vi "FILTR1.vi"() -> ()   [LabVIEW 2018]
panel:
  out "read buffer 2":string
  out "read buffer":string
  out "Postep %":dbl format="%#_2g"
  in  "START":i32=100
  in  "STOP":i32=1000
  out "XY Graph":cluster{"X":dbl[], "Y":dbl[]}[](graph)
  out "CHAN2VRMS":string
  out "CHAN1 VRMS":string
  in  "Step":i32=100
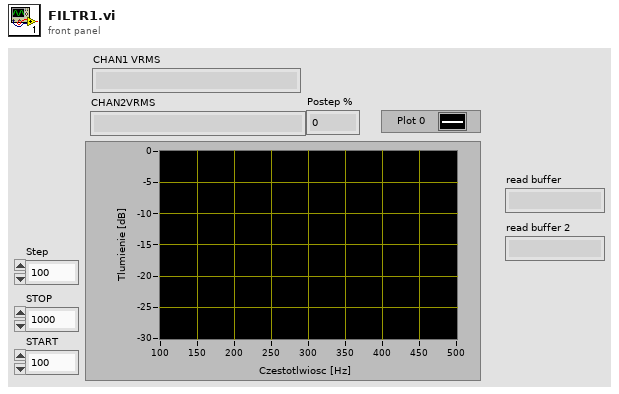
[diagram p1: front panel]
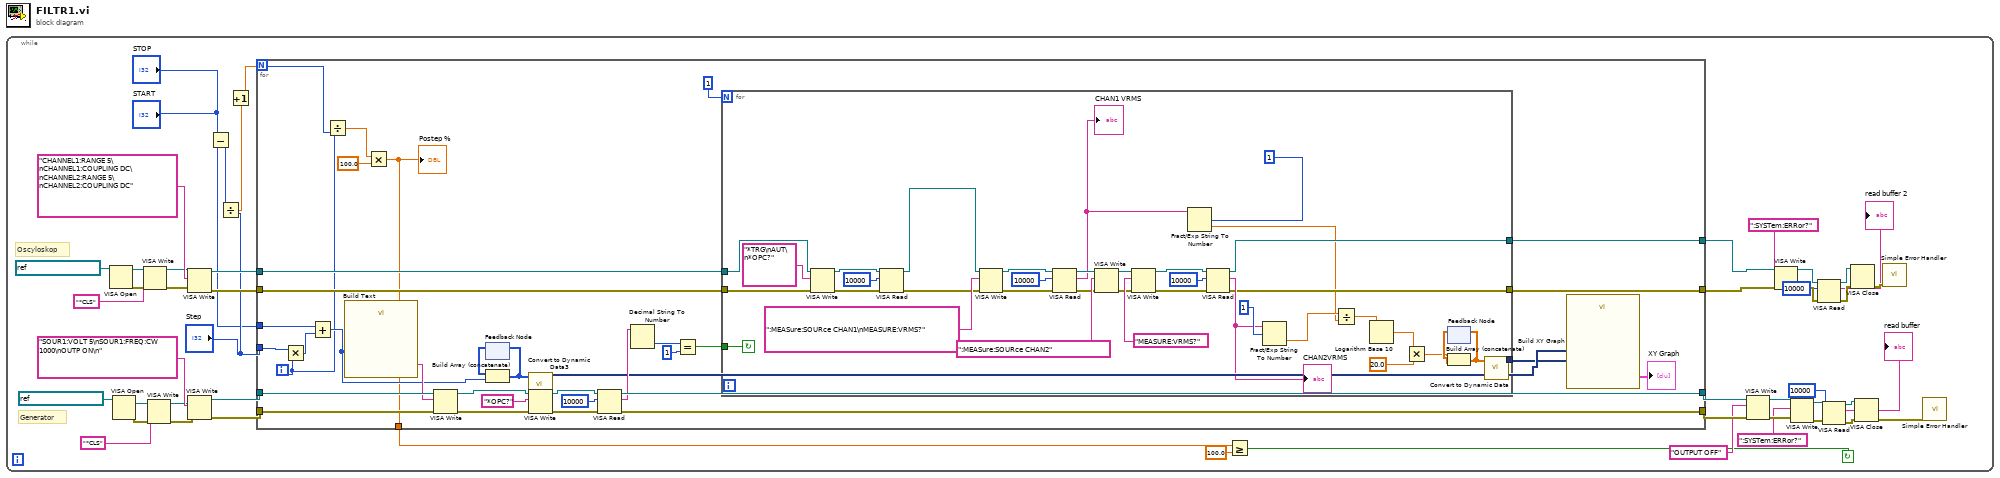
[diagram p0: block diagram]
diagram:
  n1 = while {
    stop <- w29 continue-if-true
    # "Generator"
    # "Oscyloskop"
    n2 = VISA Open(VISA resource name=refnum<visa-resource-name> "GPIB0::1::INSTR") -> (VISA resource name=w25:refnum<visa-resource-name>, error out=w28:errorcluster)  [unwired: 4 in]
    n3 = VISA Open(VISA resource name=refnum<visa-resource-name> "GPIB0::2::INSTR") -> (VISA resource name=w21:refnum<visa-resource-name>, error out=w20:errorcluster)  [unwired: 4 in]
    n4 = VISA Write(VISA resource name=w25, write buffer="*CLS", error in (no error)=w28) -> (VISA resource name out=w26:refnum<visa-resource-name>, error out=w27:errorcluster)  [unwired: 1 out]
    n5 = VISA Write(VISA resource name=w21, write buffer="*CLS", error in (no error)=w20) -> (VISA resource name out=w23:refnum<visa-resource-name>, error out=w22:errorcluster)  [unwired: 1 out]
    n6 = VISA Write(VISA resource name=w26, write buffer="CHANNEL1:RANGE 5\nCHANNEL1:COUPLING DC\nCHANNEL2:RANGE 5\nCHANNEL2:COUPLING DC", error in (no error)=w27) -> (VISA resource name out=w40:refnum<visa-resource-name>, error out=w39:errorcluster)  [unwired: 1 out]
    n7 = VISA Write(VISA resource name=w23, write buffer="SOUR1:VOLT 5\nSOUR1:FREQ:CW 1000\nOUTP ON\n", error in (no error)=w22) -> (VISA resource name out=w48:refnum<visa-resource-name>, error out=w47:errorcluster)  [unwired: 1 out]
    n8 = Subtract(x="STOP", y="START") -> (x-y=w36:i32)
    n9 = Divide(x=w36, y="Step") -> (x/y=w34:dbl)
    n10 = Increment(x=w34) -> (x+1=w35:dbl)
    n11 = for {
      N: w35 -> [w54]
      tunnel: w48 -> [w84]
      tunnel: "Step" -> [w83]
      tunnel: w47 -> [w77]
      tunnel: [w76] -> w45
      tunnel: [w75] -> w44
      tunnel: w40 -> [w69]
      tunnel: w39 -> [w68]
      tunnel: [w67] -> w15
      tunnel: [w66] -> w14
      tunnel: "START" -> [w57]
      tunnel: [w51] -> w31
      i -> [w55]
      n12 = Multiply(x=w83, y=w55) -> (x*y=w58:i32)
      n13 = Add(x=w57, y=w58) -> (x+y=w56:i32)
      n14 = Divide(x=w55, y=w54) -> (x/y=w52:dbl)
      n15 = call "Build Text"("d"=w56) -> ("Result"=w62:string)  [unwired: 13 in, 1 out]
      n16 = Multiply(x=w52, y=100.0) -> (x*y=w51:dbl)
      "Postep %" <- w51
      n17 = VISA Write(VISA resource name=w84, write buffer=w62, error in (no error)=w77) -> (VISA resource name out=w82:refnum<visa-resource-name>, error out=w79:errorcluster)  [unwired: 1 out]
      n18 = feedback #1() -> (w63:i32[])  [unwired: 1 in]
      n19 = Build Array (concatenate)(w63, w56) -> (w64:i32[])
      n20 = feedback-in #1(w64) -> ()
      n21 = call "Convert to Dynamic Data3"("Array"=w64) -> ("Dynamic Data Type"=w60:dynamicdata)  [unwired: 3 in]
      n22 = VISA Write(VISA resource name=w82, write buffer="*OPC?", error in (no error)=w79) -> (VISA resource name out=w81:refnum<visa-resource-name>, error out=w78:errorcluster)  [unwired: 1 out]
      n23 = VISA Read(VISA resource name=w81, byte count=u32 10000, error in (no error)=w78) -> (VISA resource name out=w75:refnum<visa-resource-name>, read buffer=w73:string, error out=w76:errorcluster)  [unwired: 1 out]
      n24 = Decimal String To Number(string=w73) -> (number=w72:i32)  [unwired: 2 in, 1 out]
      n25 = Equal?(x=w72, y=1) -> (x = y?=w70:bool)
      n26 = for {
        N: 1 -> [_]
        tunnel: w70 -> [w121]
        tunnel: w69 -> [w120]
        tunnel: w68 -> [w119]
        tunnel: [w104] -> w67
        tunnel: [w103] -> w66
        tunnel: [w100] -> w59
        stop <- w121 continue-if-true
        n27 = VISA Write(VISA resource name=w120, write buffer="*TRG\nAUT\n*OPC?", error in (no error)=w119) -> (VISA resource name out=w99:refnum<visa-resource-name>, error out=w96:errorcluster)  [unwired: 1 out]
        n28 = VISA Read(VISA resource name=w99, byte count=u32 10000, error in (no error)=w96) -> (VISA resource name out=w98:refnum<visa-resource-name>, error out=w97:errorcluster)  [unwired: 2 out]
        n29 = VISA Write(VISA resource name=w98, write buffer=":MEASure:SOURce CHAN1\nMEASURE:VRMS?", error in (no error)=w97) -> (VISA resource name out=w95:refnum<visa-resource-name>, error out=w94:errorcluster)  [unwired: 1 out]
        n30 = VISA Read(VISA resource name=w95, byte count=u32 10000, error in (no error)=w94) -> (VISA resource name out=w92:refnum<visa-resource-name>, read buffer=w89:string, error out=w91:errorcluster)  [unwired: 1 out]
        "CHAN1 VRMS" <- w89
        n31 = VISA Write(VISA resource name=w92, write buffer=":MEASure:SOURce CHAN2", error in (no error)=w91) -> (VISA resource name out=w108:refnum<visa-resource-name>, error out=w107:errorcluster)  [unwired: 1 out]
        n32 = VISA Write(VISA resource name=w108, write buffer="MEASURE:VRMS?", error in (no error)=w107) -> (VISA resource name out=w106:refnum<visa-resource-name>, error out=w90:errorcluster)  [unwired: 1 out]
        n33 = Fract/Exp String To Number(string=w89, offset=u32 1 ("byte count")) -> (number=w101:dbl)  [unwired: 2 in, 1 out]
        n34 = VISA Read(VISA resource name=w106, byte count=u32 10000, error in (no error)=w90) -> (VISA resource name out=w103:refnum<visa-resource-name>, read buffer=w105:string, error out=w104:errorcluster)  [unwired: 1 out]
        "CHAN2VRMS" <- w105
        n35 = Fract/Exp String To Number(string=w105, offset=u32 1 ("byte count")) -> (number=w102:dbl)  [unwired: 2 in, 1 out]
        n36 = Divide(x=w102, y=w101) -> (x/y=w88:dbl)
        n37 = Logarithm Base 10(1:w88) -> (0:w87:dbl)
        n38 = Multiply(x=w87, y=20.0) -> (x*y=w85:dbl)
        n39 = feedback #2() -> (w113:dbl[])  [unwired: 1 in]
        n40 = Build Array (concatenate)(w113, w85) -> (w114:dbl[])
        n41 = feedback-in #2(w114) -> ()
        n42 = call "Convert to Dynamic Data"("Array"=w114) -> ("Dynamic Data Type"=w100:dynamicdata)  [unwired: 3 in]
      }
      n43 = call "Build XY Graph"("Y Input"=w59, "X Input"=w60) -> ("XY Graph"=→"XY Graph":cluster{"X":dbl[], "Y":dbl[]}[])  [unwired: 8 in, 1 out]
    }
    n44 = Greater Or Equal?(x=w31, y=100.0) -> (x >= y?=w29:bool)
    n45 = VISA Write(VISA resource name=w44, write buffer="OUTPUT OFF", error in (no error)=w45) -> (VISA resource name out=w17:refnum<visa-resource-name>, error out=w18:errorcluster)  [unwired: 1 out]
    n46 = VISA Write(VISA resource name=w14, write buffer=":SYSTem:ERRor?", error in (no error)=w15) -> (VISA resource name out=w5:refnum<visa-resource-name>, error out=w4:errorcluster)  [unwired: 1 out]
    n47 = VISA Write(VISA resource name=w17, write buffer=":SYSTem:ERRor?", error in (no error)=w18) -> (VISA resource name out=w12:refnum<visa-resource-name>, error out=w11:errorcluster)  [unwired: 1 out]
    n48 = VISA Read(VISA resource name=w5, byte count=u32 10000, error in (no error)=w4) -> (VISA resource name out=w6:refnum<visa-resource-name>, read buffer=→"read buffer 2":string, error out=w3:errorcluster)  [unwired: 1 out]
    n49 = VISA Read(VISA resource name=w12, byte count=u32 10000, error in (no error)=w11) -> (VISA resource name out=w10:refnum<visa-resource-name>, read buffer=→"read buffer":string, error out=w9:errorcluster)  [unwired: 1 out]
    n50 = VISA Close(VISA resource name=w6, error in (no error)=w3) -> (error out=w38:errorcluster)
    n51 = VISA Close(VISA resource name=w10, error in (no error)=w9) -> (error out=w46:errorcluster)
    n52 = call <vilib>:"Simple Error Handler.vi"("error in (no error)"=w38) -> ()  [unwired: 4 in, 5 out]
    n53 = call <vilib>:"Simple Error Handler.vi"("error in (no error)"=w46) -> ()  [unwired: 4 in, 5 out]
  }
